vi "TestData_MySQL_InsertTextFile.vi"(6 "TXT File In":path, 7 "Ignore comment":bool, 8 "error in (no error)":errorcluster, 9 "Import Process":refnum<vi>, 10 "SQL File":path, 11 "Connection In":refnum<k7>) -> (0 "error out":errorcluster, 1 "NG?":bool, 2 "ok?":bool, 3 "ADODB._Connection Out":refnum<k7>, 4 "Result":T1)   [LabVIEW 2012, in "Lib_UEL.ATE.lvlib" / "Lib_TestData.lvlib"]
uses:
  Lib_TestData.lvlib
  <vilib>/Utility/file.llb/Read From Spreadsheet File (string).vi
  <vilib>/Utility/file.llb/Write To Spreadsheet File (string).vi
  App/Lib_App.lvlib
panel:
  out "布尔":bool
  out "Import Process":u8(slide) scale=0.0..114.0
  in  "Output Failed Record":bool
  out "Modified?":bool
  in  "Comment Signal":string
  in  "ConnectionString":T2={"IP"="localhost", "Port"="3306", "DataBase"="uel_te", "User"="root", "Password"="alpha130723"}
  out "结果字符串":string
  # "功能描述:\n- 批量插入文本数据记录到数据库.\n- 插入成功的记录, 记录前以';'注释\n- 插入失败的记录, 不注释\n- 已注释的记录, 不会进行插入数据的操作.\n- Output Failed Record开关: 失败的记录是否导出到一个单独的文件, 打开后, 输出到文件名: 原文件名+FailInsert+Date. \n- Output Failed Record: 会直接覆盖已存在的文件。"
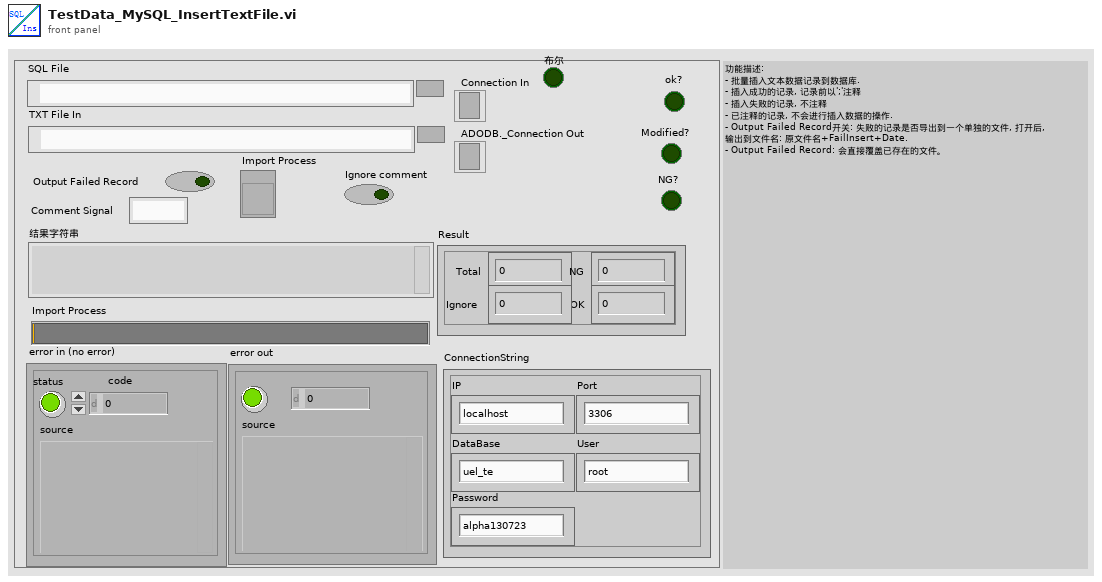
[diagram p1: front panel]
types:
  T1 = cluster{"Total":u32, "NG":u32, "OK":u32, "Ignore":u32}
  T2 = cluster{"IP":string, "Port":string, "DataBase":string, "User":string, "Password":string}
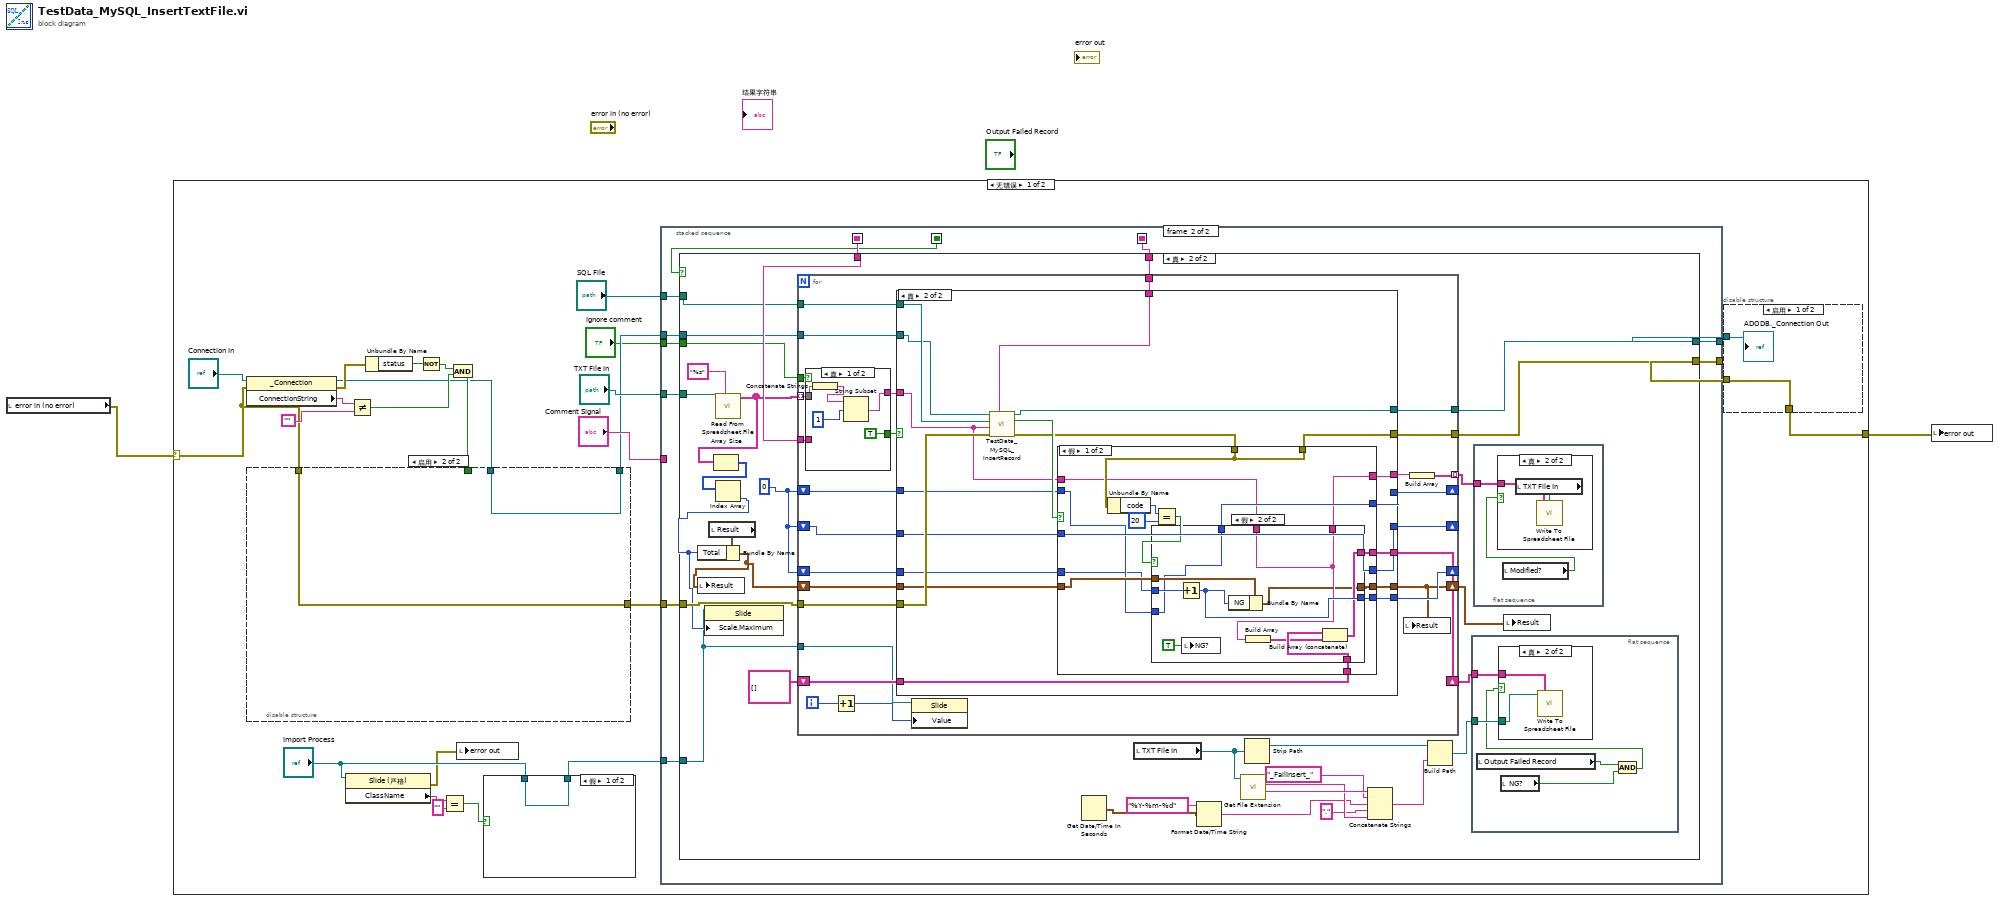
[diagram p0: block diagram]
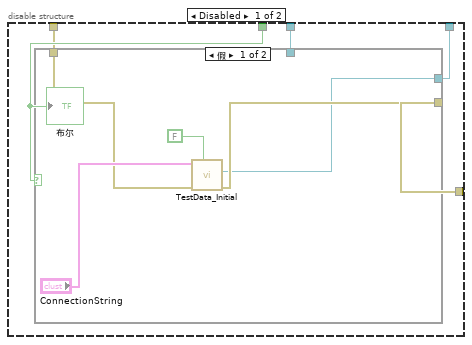
[diagram p2: hidden frame]
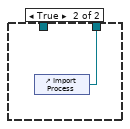
[diagram p4: hidden frame]
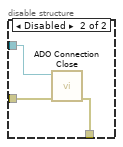
[diagram p5: hidden frame]
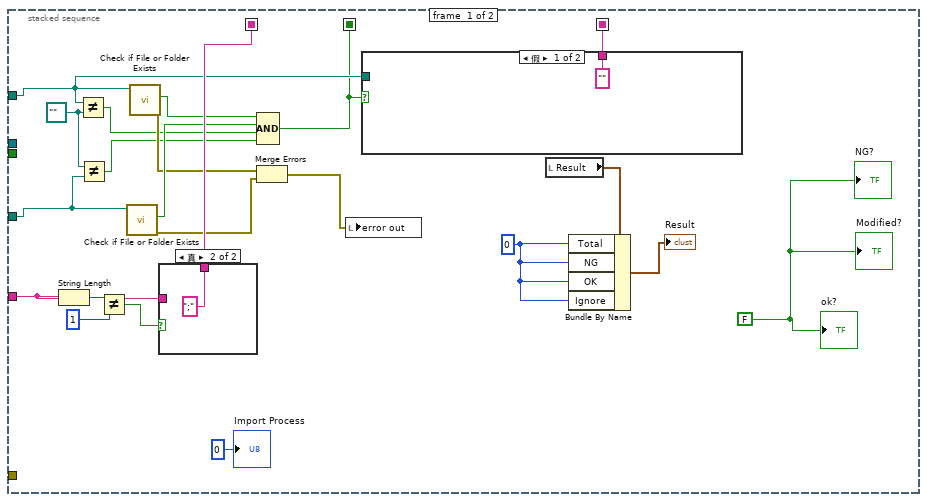
[diagram p6: hidden frame]
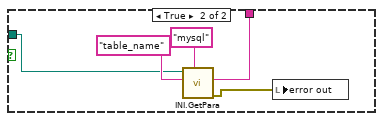
[diagram p7: hidden frame]
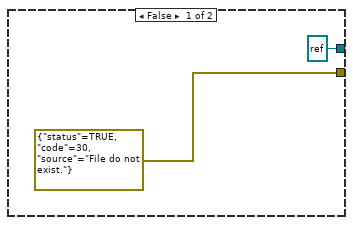
[diagram p9: hidden frame]
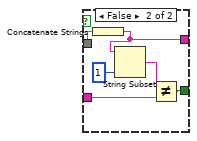
[diagram p12: hidden frame]
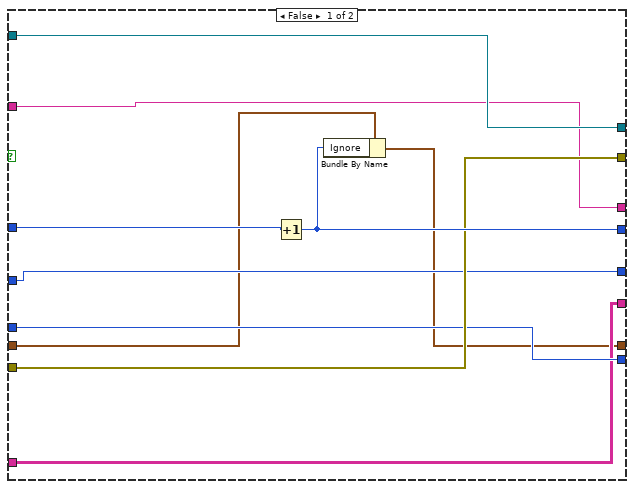
[diagram p13: hidden frame]
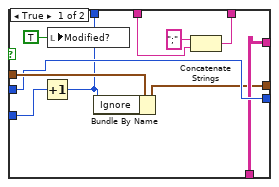
[diagram p14: hidden frame]
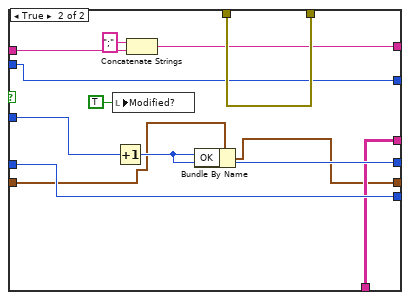
[diagram p15: hidden frame]
diagram:
  n1 = local read "error in (no error)"() -> (w1:errorcluster)
  n2 = case shown="无错误" w1 {
    selector: w1 -> [w10 w249]
    tunnel: [w11 w249] -> w2
    frame No Error {
      n3 = property class="_Connection"(reference="Connection In", error in=w10) -> (reference out=w13:refnum<k7>, error out=w18:errorcluster, "ConnectionString"=w20:string)
      n4 = property class="Slide (严格)"(reference="Import Process") -> (error out=w4:errorcluster, "ClassName"=w9:string)  [unwired: 1 in, 1 out]
      n5 = Not Equal?(x=w20, y="") -> (x != y?=w15:bool)
      n6 = Unbundle By Name(w18) -> ("status"=w17:bool)
      n7 = Not(x=w17) -> (.not. x?=w16:bool)
      n8 = Equal?(x=w9, y="") -> (x = y?=w7:bool)
      n9 = And(x=w16, y=w15) -> (x .and. y?=w14:bool)
      n10 = disable-structure shown="启用" {
        disable-tunnel: [w32 w41] -> w22
        disable-tunnel: w14 -> [w31 _]
        disable-tunnel: w13 -> [w30 w41]
        disable-tunnel: [w29 w40] -> w12
        disable-tunnel: w10 -> [w28 w40]
        frame Disabled {
          n11 = case shown="假" w31 {
            tunnel: [w33 w39] -> w32
            tunnel: w30 -> [_ w39]
            tunnel: w28 -> [w35 w38]
            tunnel: [w34 w38] -> w29
            frame False {
              n12 = call "TestData_Initial.vi"("Close Connect?"=FALSE, "error in (no error)"=w35, "ConnectionString"="ConnectionString") -> ("error out"=w34:errorcluster, "ADODB._Connection Out"=w33:refnum<k7>)  [unwired: 5 in, 2 out]
            }
            frame True {
            }
          }
          "布尔" <- w31
        }
        frame Enabled {
        }
      }
      n13 = local write "error out"(w4) -> ()
      n14 = case shown="假" w7 {
        tunnel: [w42 w43] -> w6
        tunnel: "Import Process" -> [w42 _]
        frame False {
        }
        frame True {
          n15 = control-ref of="Import Process"() -> (w43:refnum<vi>)
        }
      }
      n16 = stacked-sequence {
        seq-local: [w67 _] -> [_ w88]
        seq-local: [w50 _] -> [_ w82]
        seq-local: [w49 _] -> [_ w79]
        tunnel: w12 -> [_ w87]
        tunnel: [_ w84] -> w27
        tunnel: [_ w85] -> w23
        tunnel: "SQL File" -> [w51 w86]
        tunnel: "TXT File In" -> [w55 w89]
        tunnel: "Comment Signal" -> [w66 _]
        tunnel: w22 -> [_ w83]
        tunnel: w6 -> [_ w81]
        tunnel: "Ignore comment" -> [_ w80]
        frame #0 {
          w54 = path "" ("y")
          w63 = u32 0 ("Total")
          w62 = FALSE ("ok?")
          n17 = String Length(string=w66) -> (length=w70:i32)
          n18 = Not Equal?(x=w51, y=w54) -> (x != y?=w56:bool)
          n19 = Not Equal?(x=w54, y=w55) -> (x != y?=w53:bool)
          n20 = Not Equal?(x=w70, y=1) -> (x != y?=w68:bool)
          n21 = call <vilib>:"Check if File or Folder Exists.vi"("path"=w55) -> ("error out"=w58:errorcluster, "file or folder exists?"=w60:bool)  [unwired: 8 in, 1 out]
          n22 = call <vilib>:"Check if File or Folder Exists.vi"("path"=w51) -> ("error out"=w59:errorcluster, "file or folder exists?"=w61:bool)  [unwired: 8 in, 1 out]
          n23 = case shown="真" w68 {
            tunnel: [w77 ";"] -> w67
            tunnel: w66 -> [w77 _]
            frame False {
            }
            frame True {
            }
          }
          n24 = Compound Arithmetic op=AND(w61, w60, w56, w53) -> (w50:bool)
          n25 = Merge Errors(w59, w58) -> (w57:errorcluster)
          n26 = local write "error out"(w57) -> ()
          n27 = case shown="假" w50 {
            tunnel: w51 -> [_ w74]
            tunnel: ["" ("Para out") w72] -> w49
            frame False {
            }
            frame True {
              n28 = call "INI.GetPara.vi"("section"="mysql", "Spec_name"="table_name", "INI_File"=w74) -> ("error out"=w73:errorcluster, "Para out"=w72:string)  [unwired: 6 in, 1 out]
              n29 = local write "error out"(w73) -> ()
            }
          }
          n30 = local read "Result"() -> (w65:T1)
          n31 = Bundle By Name(cluster=w65, "Total"=w63, "NG"=w63, "OK"=w63, "Ignore"=w63) -> (→"Result":T1)
          "ok?" <- w62
          "Modified?" <- w62
          "NG?" <- w62
          "Import Process" <- u8 0 ("Import Process")
        }
        frame #1 {
          n32 = case shown="真" w82 {
            tunnel: w89 -> [_ w123]
            tunnel: w88 -> [_ w121]
            tunnel: w87 -> [_ w96]
            tunnel: w86 -> [_ w117]
            tunnel: [errorcluster {"status"=TRUE, "code"=30, "source"="File do not exist."} ("error out") w116] -> w85
            tunnel: [refnum<k7> refnum ("ADODB._Connection Out") w115] -> w84
            tunnel: w83 -> [_ w114]
            tunnel: w81 -> [_ w94]
            tunnel: w80 -> [_ w93]
            tunnel: w79 -> [_ w92]
            frame False {
            }
            frame True {
              w118 = 0
              n33 = local read "Result"() -> (w113:T1)
              n34 = call-poly <vilib>:"Read From Spreadsheet File.vi"("format (%s)"="%s", "file path (dialog if empty)"=w123) -> ("all rows"=w120:string[][])  [unwired: 5 in, 4 out]
              n35 = Array Size(array=w120) -> (size(s)=w119:i32[])
              n36 = Index Array(array=w119) -> (element=w95:i32)  [unwired: 1 in]
              n37 = Bundle By Name(cluster=w113, "Total"=w95) -> (w112:T1)
              n38 = local write "Result"(w112) -> ()
              n39 = property class="Slide"(reference=w94, "Scale.Maximum"=w95) -> ()  [unwired: 1 in, 2 out]
              n40 = for {
                tunnel: w120 -> [w160] mode=indexing
                tunnel: w121 -> [w159]
                shift-right: [w156] -> _
                shift-left: w118 -> [w157]
                shift-right: [w148] -> _
                shift-left: w118 -> [w149]
                shift-right: [w147] -> _
                shift-left: w118 -> [w146]
                tunnel: w96 -> [w155]
                tunnel: w117 -> [w153]
                tunnel: [w152] -> w116
                tunnel: [w151] -> w115
                tunnel: w114 -> [w150]
                tunnel: [w143] -> w111 mode=indexing
                shift-right: [w141] -> w109
                shift-left: string[][] [] -> [w142]
                shift-right: [w140] -> w97
                shift-left: w112 -> [w145]
                tunnel: w94 -> [w137]
                tunnel: w93 -> [w136]
                tunnel: w92 -> [w135]
                i -> [w139]
                n41 = case shown="真" w136 {
                  tunnel: w160 -> [w165 w171]
                  tunnel: w159 -> [_ w168]
                  tunnel: [TRUE w167] -> w158
                  tunnel: [w162 w166] -> w154
                  frame True {
                    n42 = Concatenate Strings(w165) -> (w164:string)
                    n43 = String Subset(string=w164, offset (0)=1 ("长度（剩余）")) -> (substring=w162:string)  [unwired: 1 in]
                  }
                  frame False {
                    n44 = Concatenate Strings(w171) -> (w166:string)
                    n45 = String Subset(string=w166, length (rest)=1 ("长度（剩余）")) -> (substring=w169:string)  [unwired: 1 in]
                    n46 = Not Equal?(x=w169, y=w168) -> (x != y?=w167:bool)
                  }
                }
                n47 = Increment(x=w139) -> (x+1=w138:i32)
                n48 = case shown="真" w158 {
                  tunnel: w157 -> [w181 w189]
                  tunnel: [w180 w188] -> w156
                  tunnel: w155 -> [w179 w201]
                  tunnel: w154 -> [w174 w187]
                  tunnel: w153 -> [_ w200]
                  tunnel: [w179 w191] -> w152
                  tunnel: [w178 w199] -> w151
                  tunnel: w150 -> [w178 w198]
                  tunnel: w149 -> [w177 w196]
                  tunnel: [w177 w195] -> w148
                  tunnel: [w176 w194] -> w147
                  tunnel: w146 -> [w176 w193]
                  tunnel: w145 -> [w175 w192]
                  tunnel: [w174 w186] -> w144
                  tunnel: [w173 w185] -> w141
                  tunnel: w142 -> [w173 w184]
                  tunnel: [w172 w183] -> w140
                  tunnel: w135 -> [_ w182]
                  frame False {
                    n49 = Increment(x=w181) -> (x+1=w180:i32)
                    n50 = Bundle By Name(cluster=w175, "Ignore"=w180) -> (w172:T1)
                  }
                  frame True {
                    n51 = call "TestData_MySQL_InsertRecord.vi"("TableName"=w182, "error in (no error)"=w201, "data_input"=w187, "SQL File"=w200, "Connection In"=w198) -> ("error out"=w190:errorcluster, "ok?"=w197:bool, "ADODB._Connection Out"=w199:refnum<k7>)  [unwired: 4 in]
                    n52 = case shown="假" w197 {
                      tunnel: w196 -> [w216 w248]
                      tunnel: [w216 w247] -> w195
                      tunnel: [w215 w246] -> w194
                      tunnel: w193 -> [w208 w246]
                      tunnel: w192 -> [w214 w245]
                      tunnel: [w213 w244] -> w191
                      tunnel: w190 -> [w213 w244]
                      tunnel: w189 -> [w209 w243]
                      tunnel: [w207 w243] -> w188
                      tunnel: w187 -> [w206 w242]
                      tunnel: [w205 w240] -> w186
                      tunnel: [w204 w238] -> w185
                      tunnel: w184 -> [w203 w238]
                      tunnel: [w202 w237] -> w183
                      frame False {
                        n53 = Unbundle By Name(w213) -> ("code"=w212:i32)
                        n54 = Equal?(x=w212, y=20) -> (x = y?=w210:bool)
                        n55 = case shown="假" w210 {
                          tunnel: w208 -> [w224 w236]
                          tunnel: [w224 w235] -> w215
                          tunnel: w214 -> [w226 w234]
                          tunnel: w209 -> [w225 w233]
                          tunnel: [w223 w233] -> w207
                          tunnel: w206 -> [w221 w231]
                          tunnel: [w220 w231] -> w205
                          tunnel: [w218 w229] -> w204
                          tunnel: w203 -> [w218 w232]
                          tunnel: [w217 w228] -> w202
                          frame True {
                            n56 = Increment(x=w225) -> (x+1=w223:i32)
                            n57 = local write "Modified?"(TRUE ("Modified?")) -> ()
                            n58 = Bundle By Name(cluster=w226, "Ignore"=w223) -> (w217:T1)
                            n59 = Concatenate Strings(";" ("字符串"), w221) -> (w220:string)
                          }
                          frame False {
                            n60 = Increment(x=w236) -> (x+1=w235:i32)
                            n61 = local write "NG?"(TRUE ("NG?")) -> ()
                            n62 = Bundle By Name(cluster=w234, "NG"=w235) -> (w228:T1)
                            n63 = Build Array(w231) -> (w230:string[])
                            n64 = Build Array (concatenate)(w232, w230) -> (w229:string[][])
                          }
                        }
                      }
                      frame True {
                        n65 = local write "Modified?"(TRUE ("Modified?")) -> ()
                        n66 = Increment(x=w248) -> (x+1=w247:i32)
                        n67 = Concatenate Strings(";" ("字符串"), w242) -> (w240:string)
                        n68 = Bundle By Name(cluster=w245, "OK"=w247) -> (w237:T1)
                      }
                    }
                  }
                }
                n69 = property class="Slide"(reference=w137, "Value"=w138) -> ()  [unwired: 1 in, 2 out]
                n70 = local write "Result"(w140) -> ()
                n71 = Build Array(w144) -> (w143:string[])
              }
              n72 = Get Date/Time In Seconds() -> (seconds since 1Jan1904=w102:timestamp)
              n73 = local read "TXT File In"() -> (w107:path)
              n74 = Format Date/Time String(time format string (%c)="%Y-%m-%d" ("时间格式字符串(%c)"), seconds (now)=w102) -> (date/time string=w100:string)  [unwired: 1 in]
              n75 = call <vilib>:"Get File Extension.vi"("file"=w107) -> ("filename without extension"=w106:string, "lowercase file extension"=w105:string)  [unwired: 7 in, 2 out]
              n76 = Strip Path(path=w107) -> (stripped path=w108:path)  [unwired: 1 out]
              n77 = Concatenate Strings(w106, "_FailInsert_" ("字符串"), w100, "." ("字符串"), w105) -> (w99:string)
              n78 = Build Path(base path=w108, name or relative path=w99) -> (appended path=w98:path)
              n79 = flat-sequence {
                tunnel: w109 -> [w128]
                tunnel: w98 -> [w127]
                frame #0 {
                  n80 = local read "Output Failed Record"() -> (w126:bool)
                  n81 = local read "NG?"() -> (w125:bool)
                  n82 = And(x=w126, y=w125) -> (x .and. y?=w124:bool)
                  n83 = case shown="真" w124 {
                    tunnel: w128 -> [_ w130]
                    tunnel: w127 -> [_ w129]
                    frame False {
                    }
                    frame True {
                      n84 = call-poly <vilib>:"Write To Spreadsheet File.vi"("2D data"=w130, "file path (dialog if empty)"=w129) -> ()  [unwired: 6 in, 1 out]
                    }
                  }
                }
              }
              n85 = flat-sequence {
                tunnel: w111 -> [w132]
                frame #0 {
                  n86 = local read "Modified?"() -> (w131:bool)
                  n87 = case shown="真" w131 {
                    tunnel: w132 -> [_ w133]
                    frame False {
                    }
                    frame True {
                      n88 = local read "TXT File In"() -> (w134:path)
                      n89 = call-poly <vilib>:"Write To Spreadsheet File.vi"("2D data"=w133, "file path (dialog if empty)"=w134) -> ()  [unwired: 6 in, 1 out]
                    }
                  }
                }
              }
              n90 = local write "Result"(w97) -> ()
            }
          }
        }
      }
      n91 = disable-structure shown="启用" {
        disable-tunnel: w27 -> [w45 w48]
        disable-tunnel: w23 -> [w44 w47]
        disable-tunnel: [w44 w46] -> w11
        frame Enabled {
          "ADODB._Connection Out" <- w45
        }
        frame Disabled {
          n92 = call <userlib>:"ADO Connection Close.vi"("error in (no error)"=w47, "ADODB._Connection In"=w48) -> ("error out"=w46:errorcluster)  [unwired: 8 in, 1 out]
        }
      }
    }
    frame Error {
    }
  }
  n93 = local write "error out"(w2) -> ()
